vi "Evaluate.vi"(0 "object in":refnum<class "PassDistance.lvclass">, 1 "Game":refnum<class "Game.lvclass">, 2 "Point":dbl[](array[numeric]), 3 "Ally?":bool, 5 "error in (no error)":errorcluster) -> (14 "object out":refnum<class "PassDistance.lvclass">, 16 "Evaluation":dbl, 19 "error out":errorcluster)   [LabVIEW 2023, in "PassDistance.lvclass"]
uses:
  PassDistance.lvclass
  PassDistance.lvclass/PassDistance.ctl
  Utilities_class/Utilities.lvclass
  Game_class/Game.lvclass
  Ball_class/Ball.lvclass
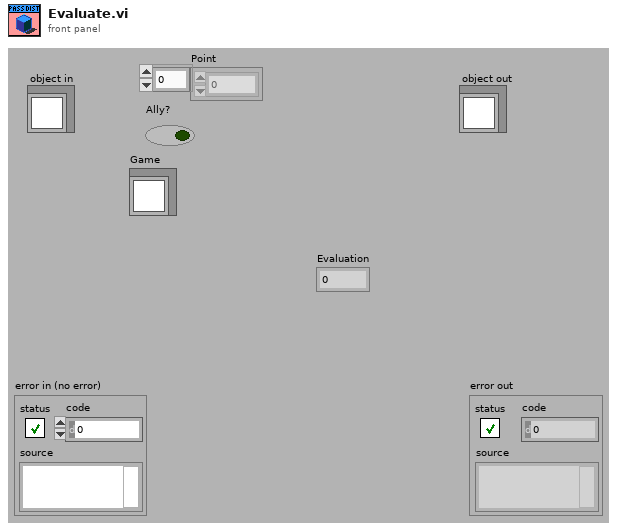
[diagram p1: front panel]
types:
  T1 = typedef "STPParameters.ctl" = cluster{"Skills":T2, "TestSkill":T4, "Events":cluster{"distanceToBallPossession":dbl, "timeForPossessionThreshold":dbl}, "Criteria":cluster{"OpenAngleToGoal":cluster{"minAngle":dbl, "maxAngle":dbl, "minEvaluation":dbl}, "PassDistance":cluster{"maxDistance":dbl, "minDistance":dbl}, "ShotTime":cluster{"shotSpeed":dbl, "keeperSpeed":dbl, "maxShotDistance":dbl, "minEvaluation":dbl}, "OneTouchShot":cluster{"MaxAngle":dbl, "minEvaluation":dbl}}}
  T2 = typedef "Skills.ctl" = cluster{"CirculateBall":T3, "ProtectBall":cluster{"DistanceFromBall":dbl}}
  T3 = typedef "CIrculateSkillParameters.ctl" = cluster{"rotationAngle":dbl, "velocityFactor":dbl, "OrientationFactor":dbl}
  T4 = typedef "TestSkills.ctl" = enum16{"AlignSkill", "PassSkill", "CirculateBall", "OneTouchShotSkill", "KickToSkill_v2", "ShootSkill", "InterceptBall", "GoToSkill_v2"}
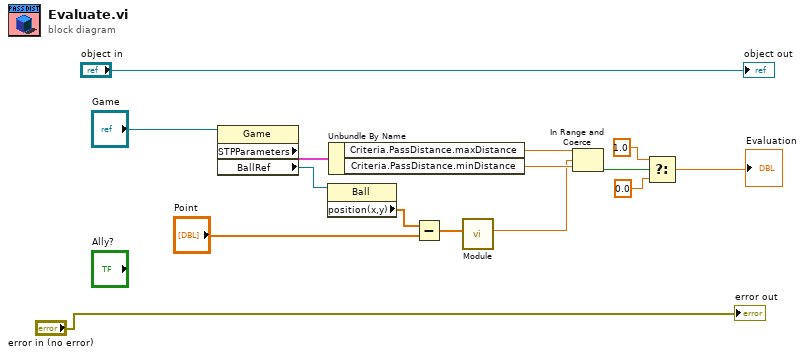
[diagram p0: block diagram]
diagram:
  n1 = property class="Game"(reference="Game") -> ("STPParameters"=w12:T1, "BallRef"=w11:refnum<class "Ball.lvclass">)  [unwired: 1 in, 2 out]
  n2 = property class="Ball"(reference=w11) -> ("position(x,y)"=w10:dbl[])  [unwired: 1 in, 2 out]
  n3 = Unbundle By Name(w12) -> ("Criteria.PassDistance.maxDistance"=w7:dbl, "Criteria.PassDistance.minDistance"=w6:dbl)
  n4 = Subtract(x=w10, y="Point") -> (x-y=w8:dbl[])
  n5 = call "Module.vi"("2D vector"=w8) -> ("Modulo"=w5:dbl)  [unwired: 8 in, 2 out]
  n6 = In Range and Coerce(upper limit=w7, x=w5, lower limit=w6) -> (In Range?=w2:bool)  [unwired: 1 out]
  n7 = Select(t=1.0, s=w2, f=0.0) -> (s? t:f=→"Evaluation":dbl)
  "error out" <- "error in (no error)"
  "object out" <- "object in"
